vi "Begin.vi"(11 "Image Size":T1=enum."160x120") -> (0 "error out":errorcluster)   [LabVIEW 2012]
doc: "Called before other user functions, this VI is expected to open initial I/O refnums, load in file data, and do all program initialization. Notice that the <B>error out</B> terminal is simply used for data flow. Wiring it to other structures or subVIs ensures that this VI runs first."
uses:
  <vilib>/Rock Robotics/WPI/Camera/WPI_CameraImageSize.ctl
  <vilib>/Rock Robotics/WPI/Camera/WPI_CameraWhite Balance Values.ctl
  <vilib>/Rock Robotics/WPI/Camera/WPI_CameraExposure Values.ctl
  <vilib>/Rock Robotics/WPI/Camera/WPI_CameraFrameRate.ctl
  <vilib>/Rock Robotics/WPI/DriverStation/WPI_DriverStationRobotMode2.ctl
  <vilib>/Rock Robotics/WPI/Joystick/WPI_JoystickDeviceEnum.ctl
  <vilib>/Rock Robotics/SystemInterfaces/DIO/FPGA_DIOPWMChannel.ctl
  <vilib>/Rock Robotics/SystemInterfaces/Typedef/FPGA_TypedefAnalogModuleForGyro.ctl
  <vilib>/Rock Robotics/SystemInterfaces/AI/FPGA_AIGyroChannel.ctl
  <vilib>/Rock Robotics/WPI/Solenoid/WPI_SolenoidChannel.ctl
  <vilib>/Rock Robotics/SystemInterfaces/DIO/FPGA_DIORelayChannel.ctl
  <vilib>/Rock Robotics/SystemInterfaces/DIO/FPGA_DIOChannel.ctl
  <vilib>/Rock Robotics/SystemInterfaces/Typedef/FPGA_TypedefDigitalModule.ctl
  <vilib>/Rock Robotics/WPI/Encoder/WPI_EncoderType.ctl
  Robot Global Data.vi
  <vilib>/Rock Robotics/WPI/RobotDrive/WPI_RobotDriveOpen2MotorWithTalon.vi
  <vilib>/Rock Robotics/WPI/MotorControl/WPI_MotorControlOpen Talon.vi
  <vilib>/Rock Robotics/WPI/Solenoid/WPI_SolenoidOpenSingle.vi
  <vilib>/Rock Robotics/WPI/Counter/WPI_CounterDigitalInputToDigitalSource.vi
  <vilib>/Rock Robotics/WPI/MotorControl/WPI_MotorControlOpen Jaguar.vi
  <vilib>/Rock Robotics/WPI/Compressor/WPI_CompressorGetSetRefNum.vi
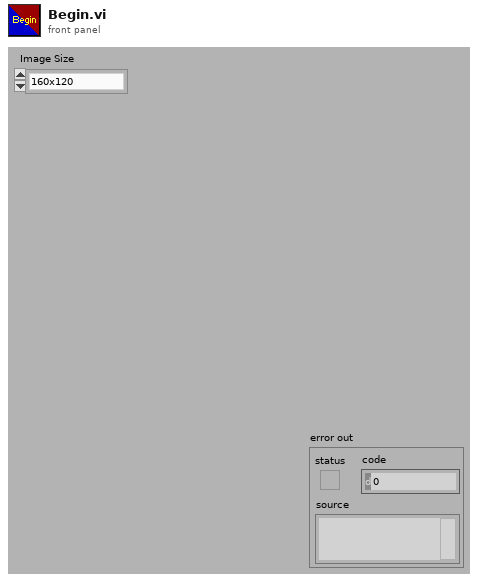
[diagram p1: front panel]
types:
  T1 = typedef "WPI_CameraImageSize.ctl" = enum16{"640x480", "320x240", "160x120"}
  T2 = typedef "FPGA_DIOPWMChannel.ctl" = enum8{"PWM 1", "PWM 2", "PWM 3", "PWM 4", "PWM 5", "PWM 6", "PWM 7", "PWM 8", "PWM 9", "PWM 10", "Invalid"}
  T3 = typedef "FPGA_TypedefDigitalModule.ctl" = enum16{"Digital Module 1", "Digital Module 2"}
  T4 = typedef "FPGA_DIORelayChannel.ctl" = enum8{"Relay 1", "Relay 2", "Relay 3", "Relay 4", "Relay 5", "Relay 6", "Relay 7", "Relay 8", "Invalid"}
  T5 = typedef "WPI_EncoderType.ctl" = enum16{"1x", "2x", "4x"}
  T6 = typedef "FPGA_DIOChannel.ctl" = enum8{"DIO 1", "DIO 2", "DIO 3", "DIO 4", "DIO 5", "DIO 6", "DIO 7", "DIO 8", "DIO 9", "DIO 10", "DIO 11", "DIO 12", "DIO 13", "DIO 14", "Invalid"}
  T7 = typedef "WPI_SolenoidChannel.ctl" = enum8{"Solenoid 1", "Solenoid 2", "Solenoid 3", "Solenoid 4", "Solenoid 5", "Solenoid 6", "Solenoid 7", "Solenoid 8", "Invalid"}
  T8 = typedef "FPGA_AIGyroChannel.ctl" = enum8{"AI 1", "AI 2", "Invalid"}
  T9 = typedef "FPGA_TypedefAnalogModuleForGyro.ctl" = enum16{"Analog Module 1"}
  T10 = typedef "WPI_JoystickDeviceEnum.ctl" = enum16{"USB 1", "USB 2", "USB 3", "USB 4", "Kinect 1", "Kinect 2"}
  T11 = typedef "WPI_DriverStationRobotMode2.ctl" = enum16{"Autonomous Disabled", "Autonomous Enabled", "Teleop Disabled", "Teleop Enabled", "Timeout", "Finish", "Test Disabled", "Test Enabled"}
  T12 = typedef "WPI_CameraFrameRate.ctl" = u32
  T13 = typedef "WPI_CameraExposure Values.ctl" = enum16{"Auto", "Flicker-free 50 Hz", "Flicker-free 60 Hz", "Hold current"}
  T14 = typedef "WPI_CameraWhite Balance Values.ctl" = enum16{"Auto", "Fixed indoor", "Fixed outdoor 1", "Fixed outdoor 2", "Fixed fluorescent 1", "Fixed fluorescent 2", "Hold current"}
  T15 = typedef "WPI_SolenoidDevRef.ctl" = cluster{"DevStatus":errorcluster, "Solenoid Module":T16, "Forward Solenoid Channel":T7, "Reverse Solenoid Channel":T7}
  T16 = typedef "FPGA_TypedefSolenoidModule.ctl" = enum16{"Solenoid Module 1", "Solenoid Module 2"}
  T17 = typedef "WPI_DigitalInputDevRef.ctl" = cluster{"DevStatus":errorcluster, "DIO Channel":T6, "Digital Module":T3}
  T18 = typedef "WPI_GyroDevRef.ctl" = cluster{"DevStatus":errorcluster, "Analog Module":T19, "Analog Channel":T20, "Offset":dbl, "Gain (VoltsPerDegree/Second)":dbl}
  T19 = typedef "FPGA_TypedefAnalogModule.ctl" = enum16{"Analog Module 1", "Analog Module 2"}
  T20 = typedef "FPGA_AIChannel.ctl" = enum8{"AI 1", "AI 2", "AI 3", "AI 4", "AI 5", "AI 6", "AI 7", "AI 8", "Invalid"}
  T21 = typedef "WPI_CompressorDevRef.ctl" = cluster{"DevStatus":errorcluster, "DigitalInputDevRef":T17, "RelayDevRef":T22}
  T22 = typedef "WPI_RelayDevRef.ctl" = cluster{"DevStatus":errorcluster, "Relay Channel":T4, "Digital Module":T3, "Relay Direction":T23}
  T23 = typedef "WPI_RelayDirection.ctl" = enum16{"Both directions", "Forward only", "Reverse only"}
  T24 = typedef "WPI_CameraDevRef.ctl" = cluster{"Camera Address":string, "CameraStatus":errorcluster, "Acquire Image Notifier":refnum<notifier>}
  T25 = typedef "WPI_JoystickDevRef.ctl" = cluster{"Device":T10}
  T26 = typedef "WPI_MotorControlDeviceRef.ctl" = cluster{"DeviceStatus":errorcluster, "Type":enum16{"PWM", "CAN"}, "PWM":cluster{"Digital Module":T3, "PWM Channel":T2, "DeadBand":T27}, "CAN":cluster{"Device Number":u8, "Control Mode":T28, "Semaphore":T29, "Max Vout":dbl}, "Invert":bool, "TransformRef":T30, "InvTransformRef":T30}
  T27 = typedef "WPI_PWMDeadband.ctl" = cluster{"Name":string, "maxPositivePwm":i32, "minPositivePwm":i32, "centerPwm":i32, "maxNegativePwm":i32, "minNegativePwm":i32, "angularRange":u16}
  T28 = typedef "WPI_CANJaguar_ControlMode.ctl" = enum8{"Percent VBus", "Current", "Speed", "Position", "Voltage"}
  T29 = typedef "Semaphore RefNum" = refnum<k1>
  T30 = typedef "WPI_PWMTransform_ConPane.ctl" = refnum<vi>
  T31 = typedef "FPGA_CounterEncoderSourceConvertionLVSourceType.ctl" = cluster{"DevStatus":errorcluster, "AnalogTriggerMode?":bool, "DigitalMode":cluster{"Digital Module":T3, "DIO Channel":T32}, "AnalogTriggerMode":cluster{"AnalogTriggerIndex":T33, "OutputType":T34}}
  T32 = typedef "FPGA_DIODigitalSourceChannel.ctl" = enum8{"DIO 1", "DIO 2", "DIO 3", "DIO 4", "DIO 5", "DIO 6", "DIO 7", "DIO 8", "DIO 9", "DIO 10", "DIO 11", "DIO 12", "DIO 13", "DIO 14", "Disabled"}
  T33 = typedef "FPGA_AnalogTriggerIndex.ctl" = enum8{"Trig 0", "Trig 1", "Trig 2", "Trig 3", "Trig 4", "Trig 5", "Trig 6", "Trig 7", "Invalid"}
  T34 = typedef "FPGA_AnalogTriggerOutType.ctl" = enum16{"InWindow", "TriggerState", "Rising", "Falling"}
  T35 = typedef "WPI_RobotDriveDevRef.ctl" = cluster{"DevStatus":errorcluster, "Motors[]":T26[], "Square Inputs":bool, "Max Output":dbl, "Isochronous":bool}
  T36 = typedef "WPI_EncoderDevRef.ctl" = cluster{"DevStatus":errorcluster, "EncoderIndex":T37, "CounterIndex":T38, "DistancePerCount":dbl, "Decoding Type":T5}
  T37 = typedef "FPGA_EncoderIdx.ctl" = enum8{"Enc 0", "Enc 1", "Enc 2", "Enc 3", "Invalid"}
  T38 = typedef "FPGA_CounterCtrSystemIndex.ctl" = enum8{"Ctr 0", "Ctr 1", "Ctr 2", "Ctr 3", "Ctr 4", "Ctr 5", "Ctr 6", "Ctr 7", "Invalid"}
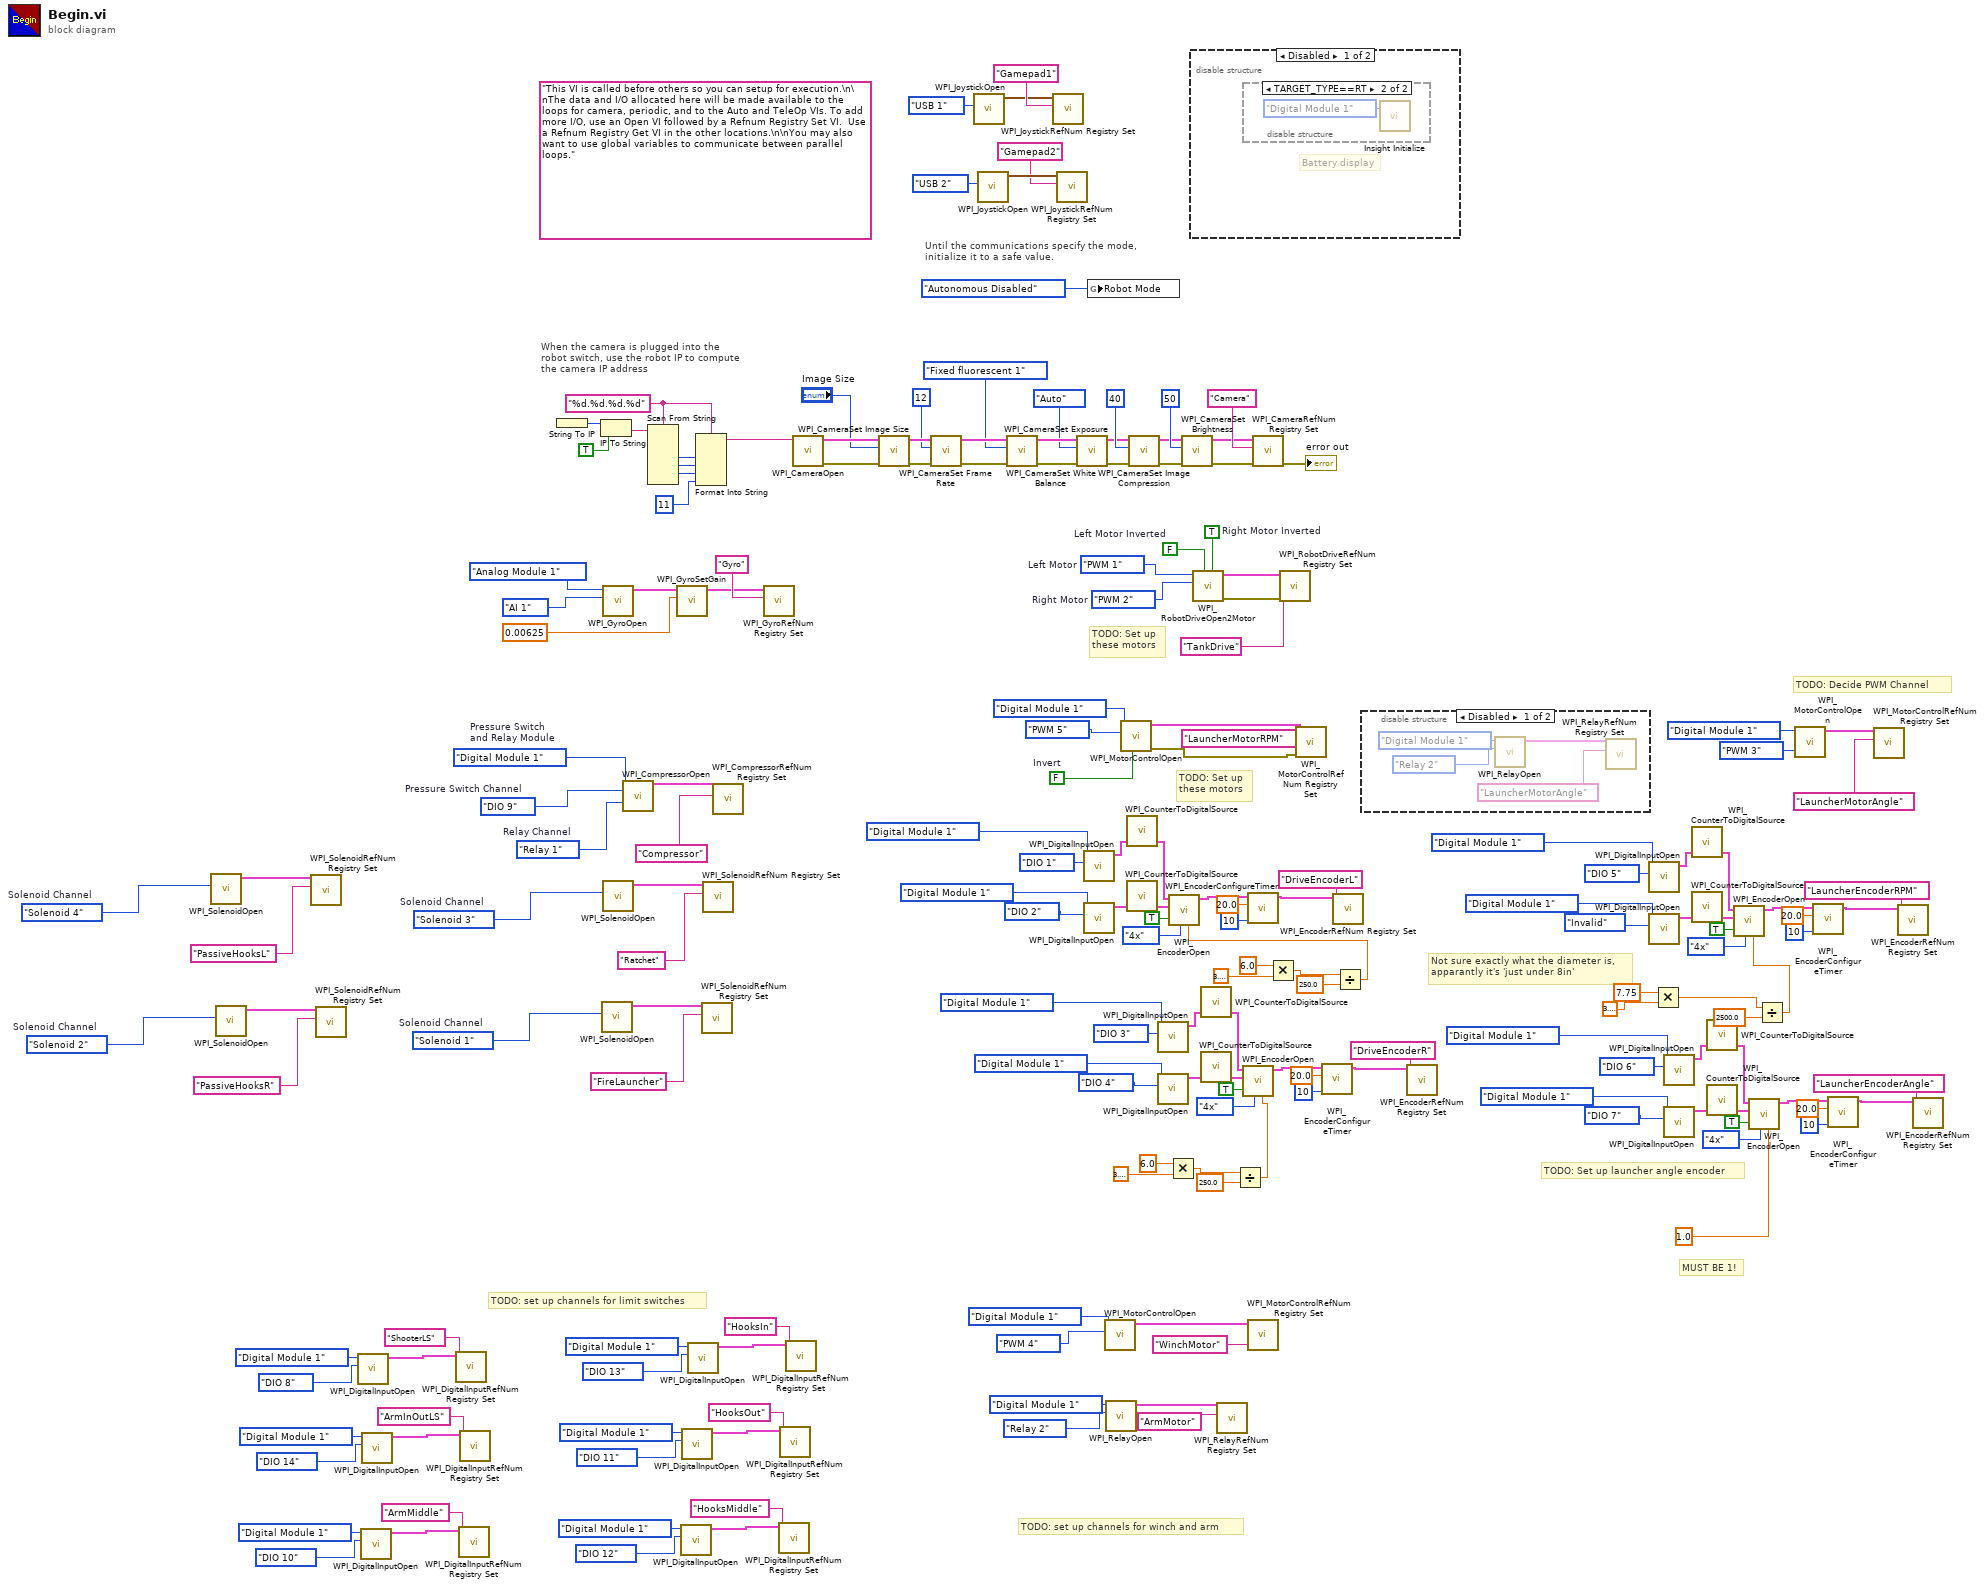
[diagram p0: block diagram]
diagram:
  w57 = WPI_SolenoidChannel."Solenoid 2"  # Solenoid Channel
  w60 = WPI_SolenoidChannel."Solenoid 4"  # Solenoid Channel
  w63 = WPI_SolenoidChannel."Solenoid 1"  # Solenoid Channel
  w127 = FPGA_TypedefDigitalModule."Digital Module 1"  # Pressure Switch and Relay Module
  w129 = FPGA_DIOChannel."DIO 9"  # Pressure Switch Channel
  w128 = FPGA_DIORelayChannel."Relay 1"  # Relay Channel
  w124 = WPI_SolenoidChannel."Solenoid 3"  # Solenoid Channel
  w137 = FALSE  # Invert
  w142 = FPGA_DIOPWMChannel."PWM 2"  # Right Motor
  w143 = FPGA_DIOPWMChannel."PWM 1"  # Left Motor
  w144 = TRUE  # Right Motor Inverted
  w145 = FALSE  # Left Motor Inverted
  w158 = "%d.%d.%d.%d" ("format string")
  (unwired) "This VI is called before others so you can setup for execution.\n\nThe data and I/O allocated here will be made available to the loops for camera, periodic, and to the Auto and TeleOp VIs. To add more I/O, use an Open VI followed by a Refnum Registry Set VI.  Use a Refnum Registry Get VI in the other locations.\n\nYou may also want to use global variables to communicate between parallel loops."
  # "MUST BE 1!"
  # "TODO: Decide PWM Channel"
  # "Not sure exactly what the diameter is, \napparantly it's 'just under 8in'"
  # "TODO: Set up launcher angle encoder"
  # "TODO: set up channels for winch and arm"
  # "TODO: set up channels for limit switches"
  # "TODO: Set up\nthese motors"
  # "TODO: Set up\nthese motors"
  # "Until the communications specify the mode,\ninitialize it to a safe value."
  # "When the camera is plugged into the\nrobot switch, use the robot IP to compute\nthe camera IP address"
  n1 = call-poly <vilib>:"WPI_SolenoidOpen.vi"("Solenoid Channel"=w60) -> ("SolenoidDevRef"=w59:T15)  [unwired: 2 in, 8 out]
  n2 = call-poly <vilib>:"WPI_SolenoidOpen.vi"("Solenoid Channel"=w57) -> ("SolenoidDevRef"=w56:T15)  [unwired: 2 in, 8 out]
  n3 = call <vilib>:"WPI_SolenoidRefNum Registry Set.vi"("refnum name"="PassiveHooksL", "SolenoidDevRef"=w59) -> ()  [unwired: 8 in, 2 out]
  n4 = call <vilib>:"WPI_SolenoidRefNum Registry Set.vi"("refnum name"="PassiveHooksR", "SolenoidDevRef"=w56) -> ()  [unwired: 8 in, 2 out]
  n5 = call <vilib>:"WPI_DigitalInputOpen.vi"("DIO Channel"=FPGA_DIOChannel."DIO 8", "Digital Module (Module 1)"=FPGA_TypedefDigitalModule."Digital Module 1") -> ("DigitalInputDevRef"=w86:T17)  [unwired: 8 in, 1 out]
  n6 = call <vilib>:"WPI_DigitalInputOpen.vi"("DIO Channel"=FPGA_DIOChannel."DIO 10", "Digital Module (Module 1)"=FPGA_TypedefDigitalModule."Digital Module 1") -> ("DigitalInputDevRef"=w102:T17)  [unwired: 8 in, 1 out]
  n7 = call <vilib>:"WPI_DigitalInputOpen.vi"("DIO Channel"=FPGA_DIOChannel."DIO 14", "Digital Module (Module 1)"=FPGA_TypedefDigitalModule."Digital Module 1") -> ("DigitalInputDevRef"=w106:T17)  [unwired: 8 in, 1 out]
  n8 = call <vilib>:"WPI_DigitalInputRefNum Registry Set.vi"("refnum name"="ShooterLS", "DigitalInputDevRef"=w86) -> ()  [unwired: 8 in, 2 out]
  n9 = call <vilib>:"WPI_DigitalInputRefNum Registry Set.vi"("refnum name"="ArmMiddle", "DigitalInputDevRef"=w102) -> ()  [unwired: 8 in, 2 out]
  n10 = call <vilib>:"WPI_DigitalInputRefNum Registry Set.vi"("refnum name"="ArmInOutLS", "DigitalInputDevRef"=w106) -> ()  [unwired: 8 in, 2 out]
  n11 = String To IP() -> (0:w165:u32)  [unwired: 1 in]
  n12 = IP To String(1:TRUE ("dot notation? (F)"), 2:w165) -> (0:w163:string)
  n13 = call-poly <vilib>:"WPI_SolenoidOpen.vi"("Solenoid Channel"=w63) -> ("SolenoidDevRef"=w62:T15)  [unwired: 2 in, 8 out]
  n14 = call <vilib>:"WPI_GyroOpen.vi"("Analog Channel"=FPGA_AIGyroChannel."AI 1", "Analog Module (Module 1)"=FPGA_TypedefAnalogModuleForGyro."Analog Module 1") -> ("GyroDevRef"=w132:T18)  [unwired: 7 in, 2 out]
  n15 = call-poly <vilib>:"WPI_SolenoidOpen.vi"("Solenoid Channel"=w124) -> ("SolenoidDevRef"=w123:T15)  [unwired: 2 in, 8 out]
  n16 = call <vilib>:"WPI_CompressorOpen.vi"("Pressure Switch Digital Module (Module 1)"=w127, "Pressure Switch DIO Channel"=w129, "Relay Channel"=w128) -> ("CompressorDevRef"=w126:T21)  [unwired: 2 in, 10 out]
  n17 = Scan From String(format string=w158, input string=w163) -> (output 1=w162:i32, output 2=w161:i32, output 3=w160:i32)  [unwired: 7 in, 3 out]
  n18 = call <vilib>:"WPI_GyroSetGain.vi"("Gain (VoltsPerDegree/Second)"=0.00625, "GyroDevRef"=w132) -> ("GyroDevRef"=w131:T18)  [unwired: 8 in, 1 out]
  n19 = call <vilib>:"WPI_DigitalInputOpen.vi"("DIO Channel"=FPGA_DIOChannel."DIO 12", "Digital Module (Module 1)"=FPGA_TypedefDigitalModule."Digital Module 1") -> ("DigitalInputDevRef"=w90:T17)  [unwired: 8 in, 1 out]
  n20 = call <vilib>:"WPI_DigitalInputOpen.vi"("DIO Channel"=FPGA_DIOChannel."DIO 11", "Digital Module (Module 1)"=FPGA_TypedefDigitalModule."Digital Module 1") -> ("DigitalInputDevRef"=w94:T17)  [unwired: 8 in, 1 out]
  n21 = call <vilib>:"WPI_DigitalInputOpen.vi"("DIO Channel"=FPGA_DIOChannel."DIO 13", "Digital Module (Module 1)"=FPGA_TypedefDigitalModule."Digital Module 1") -> ("DigitalInputDevRef"=w98:T17)  [unwired: 8 in, 1 out]
  n22 = Format Into String(format string=w158, w162, w161, w160, 11 ("Compression")) -> (resulting string=w156:string)  [unwired: 2 in, 1 out]
  n23 = call <vilib>:"WPI_SolenoidRefNum Registry Set.vi"("refnum name"="FireLauncher", "SolenoidDevRef"=w62) -> ()  [unwired: 8 in, 2 out]
  n24 = call <vilib>:"WPI_SolenoidRefNum Registry Set.vi"("refnum name"="Ratchet", "SolenoidDevRef"=w123) -> ()  [unwired: 8 in, 2 out]
  n25 = call <vilib>:"WPI_CompressorRefNum Registry Set.vi"("refnum name"="Compressor", "CompressorDevRef"=w126) -> ()  [unwired: 8 in, 2 out]
  n26 = call <vilib>:"WPI_GyroRefNum Registry Set.vi"("refnum name"="Gyro", "GyroDevRef"=w131) -> ()  [unwired: 8 in, 2 out]
  n27 = call <vilib>:"WPI_DigitalInputRefNum Registry Set.vi"("refnum name"="HooksMiddle", "DigitalInputDevRef"=w90) -> ()  [unwired: 8 in, 2 out]
  n28 = call <vilib>:"WPI_DigitalInputRefNum Registry Set.vi"("refnum name"="HooksOut", "DigitalInputDevRef"=w94) -> ()  [unwired: 8 in, 2 out]
  n29 = call <vilib>:"WPI_DigitalInputRefNum Registry Set.vi"("refnum name"="HooksIn", "DigitalInputDevRef"=w98) -> ()  [unwired: 8 in, 2 out]
  n30 = call <vilib>:"WPI_CameraOpen.vi"("Camera Address"=w156) -> ("error out"=w177:errorcluster, "CameraDevRef"=w178:T24)  [unwired: 1 in, 8 out]
  n31 = call <vilib>:"WPI_CameraSet Image Size.vi"("error in (no error)"=w177, "Image Size"="Image Size", "CameraDevRef"=w178) -> ("error out"=w176:errorcluster, "CameraDevRef Out"=w179:T24)  [unwired: 7 out]
  n32 = call <vilib>:"WPI_CameraSet Frame Rate.vi"("error in (no error)"=w176, "Frame Rate (fps)"=T12 12, "CameraDevRef"=w179) -> ("error out"=w175:errorcluster, "CameraDevRef Out"=w181:T24)  [unwired: 7 out]
  n33 = call <vilib>:"WPI_JoystickOpen.vi"("JoystickDevice"=WPI_JoystickDeviceEnum."USB 1") -> ("JoystickDevRef"=w153:T25)  [unwired: 10 in]
  n34 = call <vilib>:"WPI_JoystickOpen.vi"("JoystickDevice"=WPI_JoystickDeviceEnum."USB 2") -> ("JoystickDevRef"=w150:T25)  [unwired: 10 in]
  n35 = call <vilib>:"WPI_CameraSet White Balance.vi"("error in (no error)"=w175, "White Balance"=WPI_CameraWhite_Balance_Values."Fixed fluorescent 1", "CameraDevRef"=w181) -> ("error out"=w174:errorcluster, "CameraDevRef Out"=w180:T24)  [unwired: 7 out]
  n36 = call <vilib>:"WPI_JoystickRefNum Registry Set.vi"("refnum name"="Gamepad1", "JoystickDevRef"=w153) -> ()  [unwired: 8 in, 2 out]
  n37 = call <vilib>:"WPI_JoystickRefNum Registry Set.vi"("refnum name"="Gamepad2", "JoystickDevRef"=w150) -> ()  [unwired: 8 in, 2 out]
  n38 = call <vilib>:"WPI_CameraSet Exposure.vi"("error in (no error)"=w174, "Exposure"=WPI_CameraExposure_Values."Auto", "CameraDevRef"=w180) -> ("error out"=w173:errorcluster, "CameraDevRef Out"=w183:T24)  [unwired: 7 out]
  n39 = call <vilib>:"WPI_DigitalInputOpen.vi"("DIO Channel"=FPGA_DIOChannel."DIO 1", "Digital Module (Module 1)"=FPGA_TypedefDigitalModule."Digital Module 1") -> ("DigitalInputDevRef"=w119:T17)  [unwired: 1 in, 8 out]
  n40 = call <vilib>:"WPI_DigitalInputOpen.vi"("DIO Channel"=FPGA_DIOChannel."DIO 2", "Digital Module (Module 1)"=FPGA_TypedefDigitalModule."Digital Module 1") -> ("DigitalInputDevRef"=w120:T17)  [unwired: 1 in, 8 out]
  n41 = global write "Robot Global Data.vi" "Robot Mode"(WPI_DriverStationRobotMode2."Autonomous Disabled" ("Robot Mode")) -> ()
  n42 = call-poly <vilib>:"WPI_MotorControlOpen.vi"("PWM Channel"=FPGA_DIOPWMChannel."PWM 4", "Digital Module (Module 1)"=FPGA_TypedefDigitalModule."Digital Module 1") -> ("MotorControlDeviceRef"=w80:T26)  [unwired: 8 in, 1 out]
  n43 = call <vilib>:"WPI_RelayOpen.vi"("Relay Channel"=FPGA_DIORelayChannel."Relay 2", "Digital Module (Module 1)"=FPGA_TypedefDigitalModule."Digital Module 1") -> ("RelayDevRef"=w22:T22)  [unwired: 8 in, 1 out]
  n44 = call-poly <vilib>:"WPI_MotorControlOpen.vi"("Invert"=w137, "PWM Channel"=FPGA_DIOPWMChannel."PWM 5", "Digital Module (Module 1)"=FPGA_TypedefDigitalModule."Digital Module 1") -> ("error out"=w136:errorcluster, "MotorControlDeviceRef"=w141:T26)  [unwired: 7 in]
  n45 = call-poly <vilib>:"WPI_CounterToDigitalSource.vi"("DigitalInputDevRef"=w119) -> ("Digital Source"=w118:T31)  [unwired: 6 out]
  n46 = call-poly <vilib>:"WPI_CounterToDigitalSource.vi"("DigitalInputDevRef"=w120) -> ("Digital Source"=w121:T31)  [unwired: 6 out]
  n47 = call <vilib>:"WPI_CameraSet Image Compression.vi"("error in (no error)"=w173, "Compression"=40, "CameraDevRef"=w183) -> ("error out"=w172:errorcluster, "CameraDevRef Out"=w182:T24)  [unwired: 7 out]
  n48 = call <vilib>:"WPI_DigitalInputOpen.vi"("DIO Channel"=FPGA_DIOChannel."DIO 3", "Digital Module (Module 1)"=FPGA_TypedefDigitalModule."Digital Module 1") -> ("DigitalInputDevRef"=w76:T17)  [unwired: 1 in, 8 out]
  n49 = call <vilib>:"WPI_DigitalInputOpen.vi"("DIO Channel"=FPGA_DIOChannel."DIO 4", "Digital Module (Module 1)"=FPGA_TypedefDigitalModule."Digital Module 1") -> ("DigitalInputDevRef"=w77:T17)  [unwired: 1 in, 8 out]
  n50 = Multiply(x=6.0, y=3.141592653589793) -> (x*y=w18:dbl)
  n51 = call <vilib>:"WPI_CameraSet Brightness.vi"("error in (no error)"=w172, "Brightness"=50, "CameraDevRef"=w182) -> ("error out"=w170:errorcluster, "CameraDevRef Out"=w171:T24)  [unwired: 7 out]
  n52 = disable-structure shown="Disabled" {
    frame Disabled {
      # "Battery display"
      n53 = disable-structure shown="TARGET_TYPE==RT" {
        frame condition #0 {
        }
        frame condition #1 (active) {
          n54 = call "Insight Initialize.vi"("Digital Module"=FPGA_TypedefDigitalModule."Digital Module 1") -> ()  [unwired: 2 in]
        }
      }
    }
    frame Enabled {
    }
  }
  n55 = call-poly <vilib>:"WPI_RobotDriveOpen2Motor.vi"("Right Motor Inverted"=w144, "Left Motor Inverted"=w145, "Right Motor"=w142, "Left Motor"=w143) -> ("error out"=w146:errorcluster, "RobotDriveDevRef"=w148:T35)  [unwired: 6 in]
  n56 = call-poly <vilib>:"WPI_CounterToDigitalSource.vi"("DigitalInputDevRef"=w76) -> ("Digital Source"=w75:T31)  [unwired: 6 out]
  n57 = call-poly <vilib>:"WPI_CounterToDigitalSource.vi"("DigitalInputDevRef"=w77) -> ("Digital Source"=w78:T31)  [unwired: 6 out]
  n58 = call <vilib>:"WPI_RelayRefNum Registry Set.vi"("refnum name"="ArmMotor", "RelayDevRef"=w22) -> ()  [unwired: 8 in, 2 out]
  n59 = Divide(x=w18, y=250.0) -> (x/y=w16:dbl)
  n60 = call <vilib>:"WPI_EncoderOpen.vi"("DistancePerCount"=w16, "Decoding Type"=WPI_EncoderType."4x", "Invert Direction (False)"=TRUE, "BSource"=w78, "ASource"=w75) -> ("EncoderDevRef"=w72:T36)  [unwired: 3 in, 3 out]
  n61 = call <vilib>:"WPI_MotorControlRefNum Registry Set.vi"("refnum name"="WinchMotor", "MotorControlDevRef"=w80) -> ()  [unwired: 8 in, 2 out]
  n62 = call <vilib>:"WPI_CameraRefNum Registry Set.vi"("error in (no error)"=w170, "refnum name"="Camera", "CameraDevRef"=w171) -> ("error out"=→"error out":errorcluster)  [unwired: 8 out]
  n63 = Multiply(x=6.0, y=3.141592653589793) -> (x*y=w13:dbl)
  n64 = call <vilib>:"WPI_RobotDriveRefNum Registry Set.vi"("error in (no error)"=w146, "refnum name"="TankDrive", "RobotDriveDevRef"=w148) -> ()  [unwired: 7 in, 2 out]
  n65 = call <vilib>:"WPI_MotorControlRefNum Registry Set.vi"("error in (no error)"=w136, "refnum name"="LauncherMotorRPM", "MotorControlDevRef"=w141) -> ()  [unwired: 7 in, 2 out]
  n66 = call <vilib>:"WPI_EncoderConfigureTimer.vi"("Number Samples to Average"=u8 10, "Minimum Rate"=20.0, "EncoderDevRef"=w72) -> ("EncoderDevRef"=w69:T36)  [unwired: 1 in, 7 out]
  n67 = Divide(x=w13, y=250.0) -> (x/y=w11:dbl)
  n68 = call <vilib>:"WPI_EncoderOpen.vi"("DistancePerCount"=w11, "Decoding Type"=WPI_EncoderType."4x", "Invert Direction (False)"=TRUE, "BSource"=w121, "ASource"=w118) -> ("EncoderDevRef"=w115:T36)  [unwired: 3 in, 3 out]
  n69 = call <vilib>:"WPI_EncoderConfigureTimer.vi"("Number Samples to Average"=u8 10, "Minimum Rate"=20.0, "EncoderDevRef"=w115) -> ("EncoderDevRef"=w112:T36)  [unwired: 1 in, 7 out]
  n70 = call <vilib>:"WPI_EncoderRefNum Registry Set.vi"("refnum name"="DriveEncoderL", "EncoderDevRef"=w112) -> ()  [unwired: 8 in, 2 out]
  n71 = disable-structure shown="Disabled" {
    frame Disabled {
      n72 = call <vilib>:"WPI_RelayOpen.vi"("Relay Channel"=FPGA_DIORelayChannel."Relay 2", "Digital Module (Module 1)"=FPGA_TypedefDigitalModule."Digital Module 1") -> ("RelayDevRef"=w189:T22)  [unwired: 8 in, 1 out]
      n73 = call <vilib>:"WPI_RelayRefNum Registry Set.vi"("refnum name"="LauncherMotorAngle", "RelayDevRef"=w189) -> ()  [unwired: 8 in, 2 out]
    }
    frame Enabled {
    }
  }
  n74 = call <vilib>:"WPI_EncoderRefNum Registry Set.vi"("refnum name"="DriveEncoderR", "EncoderDevRef"=w69) -> ()  [unwired: 8 in, 2 out]
  n75 = call <vilib>:"WPI_DigitalInputOpen.vi"("DIO Channel"=FPGA_DIOChannel."DIO 5", "Digital Module (Module 1)"=FPGA_TypedefDigitalModule."Digital Module 1") -> ("DigitalInputDevRef"=w52:T17)  [unwired: 1 in, 8 out]
  n76 = call <vilib>:"WPI_DigitalInputOpen.vi"("DIO Channel"=FPGA_DIOChannel."Invalid", "Digital Module (Module 1)"=FPGA_TypedefDigitalModule."Digital Module 1") -> ("DigitalInputDevRef"=w53:T17)  [unwired: 1 in, 8 out]
  n77 = Multiply(x=7.75, y=3.141592653589793) -> (x*y=w7:dbl)
  n78 = call <vilib>:"WPI_DigitalInputOpen.vi"("DIO Channel"=FPGA_DIOChannel."DIO 6", "Digital Module (Module 1)"=FPGA_TypedefDigitalModule."Digital Module 1") -> ("DigitalInputDevRef"=w37:T17)  [unwired: 1 in, 8 out]
  n79 = call <vilib>:"WPI_DigitalInputOpen.vi"("DIO Channel"=FPGA_DIOChannel."DIO 7", "Digital Module (Module 1)"=FPGA_TypedefDigitalModule."Digital Module 1") -> ("DigitalInputDevRef"=w38:T17)  [unwired: 1 in, 8 out]
  n80 = call-poly <vilib>:"WPI_CounterToDigitalSource.vi"("DigitalInputDevRef"=w52) -> ("Digital Source"=w51:T31)  [unwired: 6 out]
  n81 = call-poly <vilib>:"WPI_CounterToDigitalSource.vi"("DigitalInputDevRef"=w53) -> ("Digital Source"=w54:T31)  [unwired: 6 out]
  n82 = call-poly <vilib>:"WPI_CounterToDigitalSource.vi"("DigitalInputDevRef"=w37) -> ("Digital Source"=w36:T31)  [unwired: 6 out]
  n83 = call-poly <vilib>:"WPI_CounterToDigitalSource.vi"("DigitalInputDevRef"=w38) -> ("Digital Source"=w39:T31)  [unwired: 6 out]
  n84 = call <vilib>:"WPI_EncoderOpen.vi"("DistancePerCount"=1.0, "Decoding Type"=WPI_EncoderType."4x", "Invert Direction (False)"=TRUE, "BSource"=w39, "ASource"=w36) -> ("EncoderDevRef"=w33:T36)  [unwired: 3 in, 3 out]
  n85 = Divide(x=w7, y=2500.0) -> (x/y=w10:dbl)
  n86 = call <vilib>:"WPI_EncoderOpen.vi"("DistancePerCount"=w10, "Decoding Type"=WPI_EncoderType."4x", "Invert Direction (False)"=TRUE, "BSource"=w54, "ASource"=w51) -> ("EncoderDevRef"=w48:T36)  [unwired: 3 in, 3 out]
  n87 = call-poly <vilib>:"WPI_MotorControlOpen.vi"("PWM Channel"=FPGA_DIOPWMChannel."PWM 3", "Digital Module (Module 1)"=FPGA_TypedefDigitalModule."Digital Module 1") -> ("MotorControlDeviceRef"=w3:T26)  [unwired: 8 in, 1 out]
  n88 = call <vilib>:"WPI_EncoderConfigureTimer.vi"("Number Samples to Average"=u8 10, "Minimum Rate"=20.0, "EncoderDevRef"=w48) -> ("EncoderDevRef"=w45:T36)  [unwired: 1 in, 7 out]
  n89 = call <vilib>:"WPI_EncoderConfigureTimer.vi"("Number Samples to Average"=u8 10, "Minimum Rate"=20.0, "EncoderDevRef"=w33) -> ("EncoderDevRef"=w30:T36)  [unwired: 1 in, 7 out]
  n90 = call <vilib>:"WPI_MotorControlRefNum Registry Set.vi"("refnum name"="LauncherMotorAngle", "MotorControlDevRef"=w3) -> ()  [unwired: 8 in, 2 out]
  n91 = call <vilib>:"WPI_EncoderRefNum Registry Set.vi"("refnum name"="LauncherEncoderRPM", "EncoderDevRef"=w45) -> ()  [unwired: 8 in, 2 out]
  n92 = call <vilib>:"WPI_EncoderRefNum Registry Set.vi"("refnum name"="LauncherEncoderAngle", "EncoderDevRef"=w30) -> ()  [unwired: 8 in, 2 out]
